vi "Change Wheel Type by Index.vi"(7 "active wheel indexes":i32[](array[numeric]), 8 "error in (no error)":errorcluster, 10 "wheel type":string, 11 "steering frame ref in":refnum<data-value>) -> (0 "error out":errorcluster, 1 "changed?":bool, 3 "steering frame ref out":refnum<data-value>)   [LabVIEW 2017, in "NI_Robotics_Configure Steering Frame.lvlib"]
uses:
  <vilib>/robotics/Dialog/Configure Steering Frame/NI_Robotics_Configure Steering Frame.lvlib
  <vilib>/robotics/Steering/Steering Frame/NI_Robotics_Steering Frame.lvclass
  <vilib>/robotics/Steering/Steering Frame/NI_Robotics_Steering Frame.lvclass/NI_Robotics_Steering Frame.ctl
  <vilib>/robotics/Steering/Wheel/NI_Robotics_Wheel.lvclass/NI_Robotics_Wheel.ctl
  <vilib>/robotics/Steering/Steering Frame/Get Multiple Wheels in Steering Frame.vi
  <vilib>/robotics/Steering/Wheel/Get General Wheel Information.vi
  <vilib>/robotics/Steering/Wheel/Get Motor Communication.vi
  <vilib>/robotics/Steering/Wheel/Get Wheel Parameters.vi
  <vilib>/robotics/Steering/Fixed Wheel/NI_Robotics_Fixed Wheel.lvclass
  c:/Program Files (x86)/National Instruments/LabVIEW 2017/vi.lib/robotics/Steering/Wheel/NI_Robotics_Wheel.lvclass
  <vilib>/robotics/Steering/Steering Wheel/NI_Robotics_Steering Wheel.lvclass
  <vilib>/robotics/Steering/Caster Wheel/NI_Robotics_Caster Wheel.lvclass
  <vilib>/robotics/Steering/Mecanum Wheel/NI_Robotics_Mecanum Wheel.lvclass
  <vilib>/robotics/Steering/Omnidirectional Wheel/NI_Robotics_Omnidirectional Wheel.lvclass
  <vilib>/robotics/Steering/Omnidirectional Wheel/Create Omnidirectional Wheel.vi
  <vilib>/robotics/Steering/Mecanum Wheel/Create Mecanum Wheel.vi
  <vilib>/robotics/Steering/Caster Wheel/Create Caster Wheel.vi
  <vilib>/robotics/Steering/Steering Wheel/Create Steering Wheel.vi
  <vilib>/robotics/Steering/Fixed Wheel/Create Fixed Wheel.vi
  <vilib>/robotics/Steering/Wheel/NI_Robotics_Wheel.lvclass
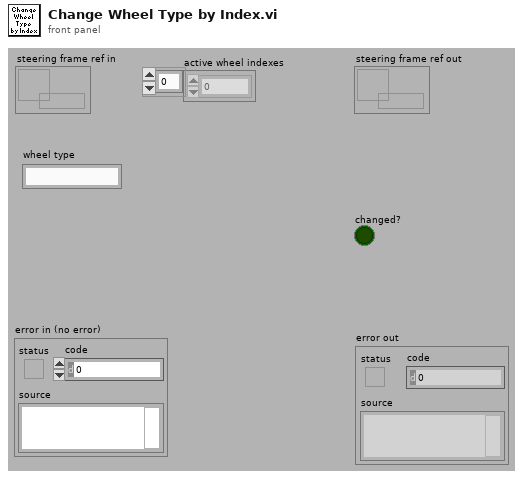
[diagram p1: front panel]
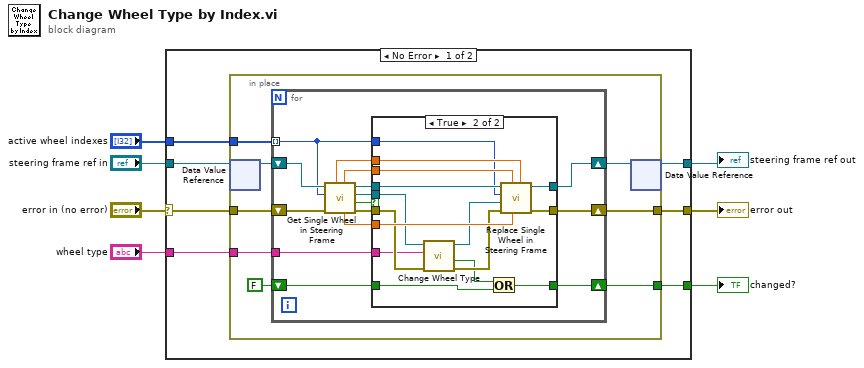
[diagram p0: block diagram]
diagram:
  n1 = case shown="No Error" "error in (no error)" {
    selector: "error in (no error)" -> [w12 w57]
    tunnel: "wheel type" -> [w14 _]
    tunnel: [w13 w57] -> w5
    tunnel: [w8 _] -> w4
    tunnel: "steering frame ref in" -> [w11 w56]
    tunnel: "active wheel indexes" -> [w9 _]
    tunnel: [w10 w56] -> w1
    frame No Error {
      n2 = in-place {
        in-place-border: w9 -> [w19]
        in-place-border: w14 -> [w22]
        in-place-border: w12 -> [w20]
        in-place-border: [w17] -> w13
        in-place-border: [w15] -> w8
        n3 = in-place-dvr #1(w11) -> (w21:refnum<class "NI_Robotics_Steering Frame.lvclass">)  [unwired: 1 out]
        n4 = for {
          tunnel: w22 -> [w37]
          tunnel: w19 -> [w28] mode=indexing
          shift-right: [w27] -> w18
          shift-left: w21 -> [w36]
          shift-right: [w26] -> w17
          shift-left: w20 -> [w33]
          shift-right: [w24] -> w15
          shift-left: FALSE -> [w23]
          n5 = call <vilib>:"Get Single Wheel in Steering Frame.vi"("error in (no error)"=w33, "wheel index"=w28, "steering frame in"=w36) -> ("error out"=w34:errorcluster, "found?"=w25:bool, "wheel"=w35:refnum<class "NI_Robotics_Wheel.lvclass">, "steering frame out"=w32:refnum<class "NI_Robotics_Steering Frame.lvclass">, "frame angle (rad)"=w29:dbl, "y position"=w31:dbl, "x position"=w30:dbl)  [unwired: 2 in]
          n6 = case shown="True" w25 {
            tunnel: w37 -> [_ w44]
            tunnel: w35 -> [_ w48]
            tunnel: w34 -> [w39 w45]
            tunnel: w32 -> [w40 w55]
            tunnel: w31 -> [_ w54]
            tunnel: w30 -> [_ w53]
            tunnel: w29 -> [_ w52]
            tunnel: w28 -> [_ w51]
            tunnel: [w40 w50] -> w27
            tunnel: [w39 w49] -> w26
            tunnel: [w38 w42] -> w24
            tunnel: w23 -> [w38 w41]
            frame False {
            }
            frame True {
              n7 = call <vilib>:"Change Wheel Type.vi"("error in (no error)"=w45, "wheel type"=w44, "wheel in"=w48) -> ("error out"=w46:errorcluster, "changed?"=w43:bool, "wheel out"=w47:refnum<class "NI_Robotics_Wheel.lvclass">)  [unwired: 6 in]
              n8 = Or(x=w43, y=w41) -> (x .or. y?=w42:bool)
              n9 = call <vilib>:"Replace Single Wheel in Steering Frame.vi"("x position"=w53, "frame angle (rad)"=w52, "y position"=w54, "error in (no error)"=w46, "wheel"=w47, "wheel index"=w51, "steering frame in"=w55) -> ("error out"=w49:errorcluster, "steering frame out"=w50:refnum<class "NI_Robotics_Steering Frame.lvclass">)  [unwired: 2 in, 1 out]
            }
          }
        }
        n10 = in-place-dvr #1(w18) -> (w10:refnum<data-value>)  [unwired: 1 out]
      }
    }
    frame Error {
    }
  }
  "error out" <- w5
  "changed?" <- w4
  "steering frame ref out" <- w1
